vi "IV close.vi"(8 "error in (no error)":errorcluster) -> (0 "error out":errorcluster, 3 "return type":i32)   [LabVIEW 2022 SP3, in "IVIUM_remdriver.lvlib"]
uses:
  IVIUM_remdriver.lvlib
  IVIUM_remdriver.dll
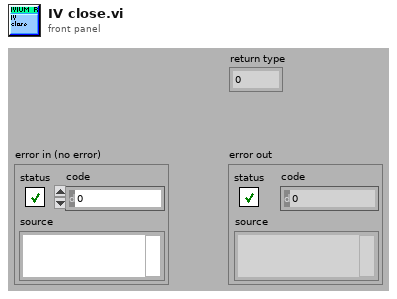
[diagram p1: front panel]
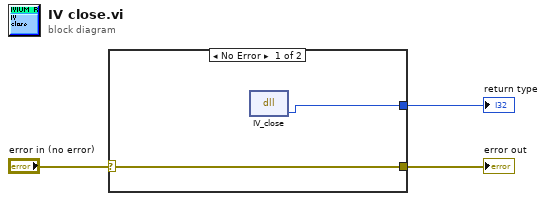
[diagram p0: block diagram]
diagram:
  n1 = case shown="No Error" "error in (no error)" {
    selector: "error in (no error)" -> [w5 w6]
    tunnel: [w5 w6] -> w2
    tunnel: [w4 _] -> w1
    frame No Error {
      n2 = dll-call lib="C:/Users/Benj/Desktop/SEC Software V4.8/Dependencies/Drivers and Aux files/IVIUM/IVIUM_remdriver.*" fn="IV_close"() -> (w4:i32)  [unwired: 3 in, 2 out]
    }
    frame Error {
    }
  }
  "return type" <- w1
  "error out" <- w2
